vi "shutterSelect.vi"(6 "Delay between send and receive [ms]":i32=100, 8 "error in (no error)":errorcluster, 10 "shutter":T1, 11 "Monochromator in":refnum<class "Monochromator.lvclass">) -> (0 "error out":errorcluster, 1 "ID":i32, 2 "results-JSON string":string, 3 "Monochromator out":refnum<class "Monochromator.lvclass">)   [LabVIEW 2023, in "Monochromator.lvclass"]
uses:
  Monochromator.lvclass
  Monochromator.lvclass/Monochromator.ctl
  7fe8abea-6ecd-46de-aa11-ce8637911b6a.vi
  GenericDevice/GenericDevice.lvclass
  <vilib>/IlluminatedG/lv-web-crypto/lv-json/JSON/JSON.lvlib
  35d46a5a-fd7c-4445-96f4-e877dae8f93b.vi
  ShutterIDEnum.ctl
panel:
  # "Connector Pane"
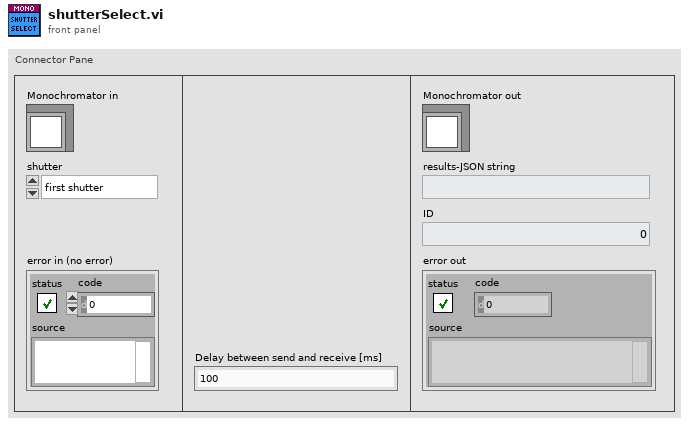
[diagram p1: front panel]
types:
  T1 = typedef "Monochromator.lvclass/ShutterIDEnum.ctl" = enum16{"first shutter", "second shutter"}
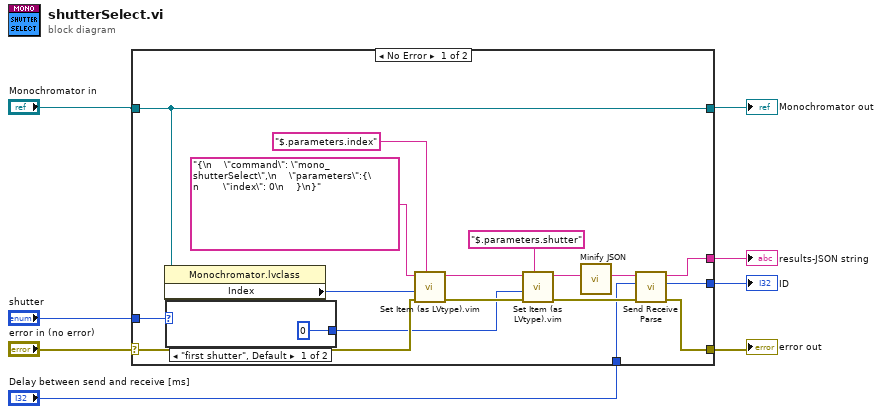
[diagram p0: block diagram]
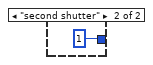
[diagram p2: hidden frame]
diagram:
  n1 = case shown="No Error" "error in (no error)" {
    selector: "error in (no error)" -> [w21 w29]
    tunnel: [w18 w29] -> w5
    tunnel: [w23 w28] -> w7
    tunnel: "Monochromator in" -> [w23 w28]
    tunnel: [w20 _] -> w3
    tunnel: [w19 _] -> w4
    tunnel: "shutter" -> [w11 _]
    tunnel: "Delay between send and receive [ms]" -> [w9 _]
    frame No Error {
      n2 = property class="Monochromator.lvclass"(reference=w23) -> ("Index"=w22:i32)  [unwired: 1 in, 2 out]
      n3 = case shown="\"first shutter\", Default" w11 {
        tunnel: [0 1] -> w10
        frame "first shutter", Default {
        }
        frame "second shutter" {
        }
      }
      n4 = call "Set Item (as LVtype).vim"("$Path or Item Name"="$.parameters.index", "error in (no error)"=w21, "Anything"=w22, "JSON"="{\n    \"command\": \"mono_shutterSelect\",\n    \"parameters\":{\n        \"index\": 0\n    }\n}") -> ("error out"=w15:errorcluster, "<JSON>"=w13:string)  [unwired: 4 in, 1 out]
      n5 = call "Set Item (as LVtype).vim"("$Path or Item Name"="$.parameters.shutter", "error in (no error)"=w15, "Anything"=w10, "JSON"=w13) -> ("error out"=w14:errorcluster, "<JSON>"=w12:string)  [unwired: 4 in, 1 out]
      n6 = call <vilib>:"Minify JSON.vi"("JSON String"=w12) -> ("Minified JSON"=w17:string)  [unwired: 10 in]
      n7 = call "Send Receive Parse.vi"("error in"=w14, "Delay between send and receive [ms]"=w9, "<JSON>"=w17) -> ("error out"=w18:errorcluster, "ID"=w19:i32, "results-JSON string"=w20:string)  [unwired: 6 in]
    }
    frame Error {
    }
  }
  "error out" <- w5
  "Monochromator out" <- w7
  "ID" <- w4
  "results-JSON string" <- w3
